vi "lua_getfield.vi"(8 "error in (no error)":errorcluster, 9 "field":string, 10 "index":i32, 11 "lua_state_p":u64) -> (0 "error out":errorcluster, 2 "lua type":T1 items=["LUA_TNONE"=-1, "LUA_TNIL"=0, "LUA_TBOOLEAN"=1, "LUA_TLIGHTUSERDATA"=2, "LUA_TNUMBER"=3, "LUA_TSTRING"=4, "LUA_TTABLE"=5, "LUA_TFUNCTION"=6, "LUA_TUSERDATA"=7, "LUA_TTHREAD"=8, "LUA_NUMTYPES"=9], 3 "lua_state_p out":u64)   [LabVIEW 2020, in "lua.dll.lvlib"]
uses:
  lua_types.ctl
  lua.dll.lvlib
  lua54.dll
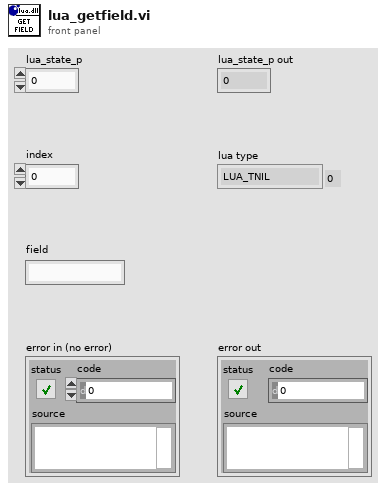
[diagram p1: front panel]
types:
  T1 = typedef "lua.dll.lvlib/lua_types.ctl" = i32
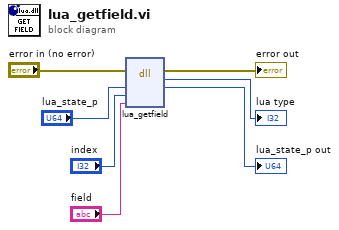
[diagram p0: block diagram]
diagram:
  n1 = dll-call lib="C:/Users/Nicholas Folse/Documents/workspace/github-tauterra.llc/Lua for LabVIEW/lib/lua.dll/lua54**.*" fn="lua_getfield"(error in="error in (no error)", "lua_state_p"="lua_state_p", "index"="index", "field"="field") -> (error out=→"error out":errorcluster, "type"=→"lua type":i32, "lua_state_p"=→"lua_state_p out":u64)  [unwired: 4 in, 1 out]
